vi "AuMT8852B Path Offset Table Read.vi"(5 "Frequency units (Channel)":enum16{"Channel", "MHz"}(ring), 7 "Table (1)":i32=1, 8 "error in (no error)":errorcluster, 11 "VISA session":refnum<visa-resource-name>) -> (0 "error out":errorcluster, 2 "error code":i32, 3 "VISA session out":refnum<visa-resource-name>, 4 "Table values":dbl[][](array[numeric]) format="%.2f")   [LabVIEW 2017]
doc: "Anritsu MT8852B Bluetooth Tester\n\nRetrieves all frequency/offset pairs in a table.\n\nINPUTS\nTable - path offset table (1-10) to use.\nFrequency units - whether the frequencies will be returned as channels or as frequencies in MHz.\n\nOUTPUTS\nTable values - two-dimensional array containing all table frequencies and offsets."
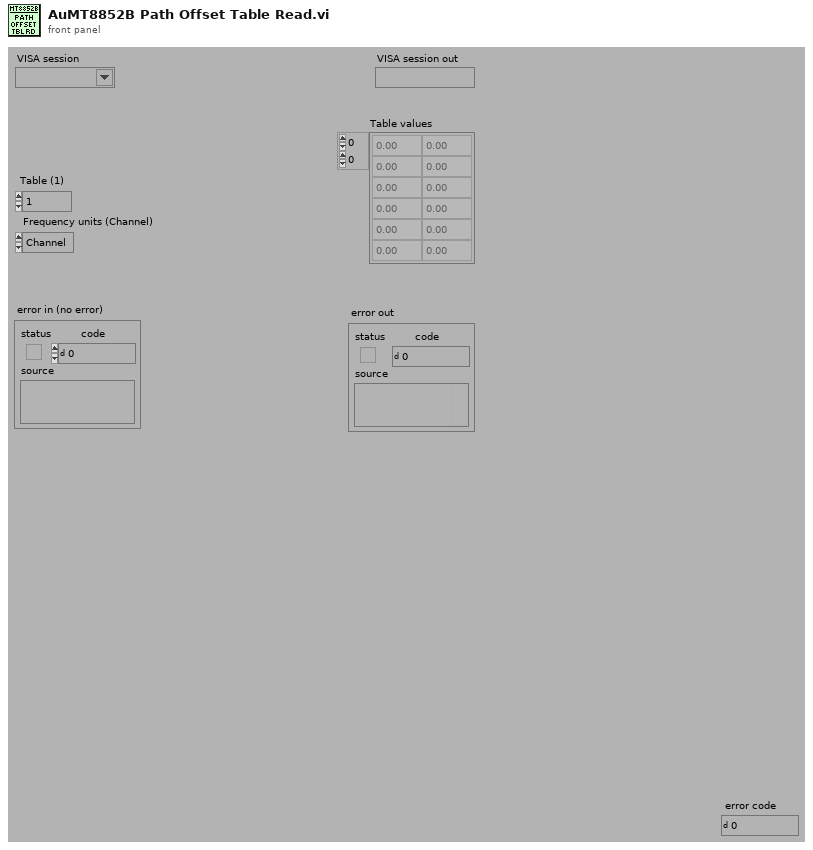
[diagram p1: front panel]
types:
  T1 = enum16{"Simulate", "Range check", "Cache", "Query instrument status"}
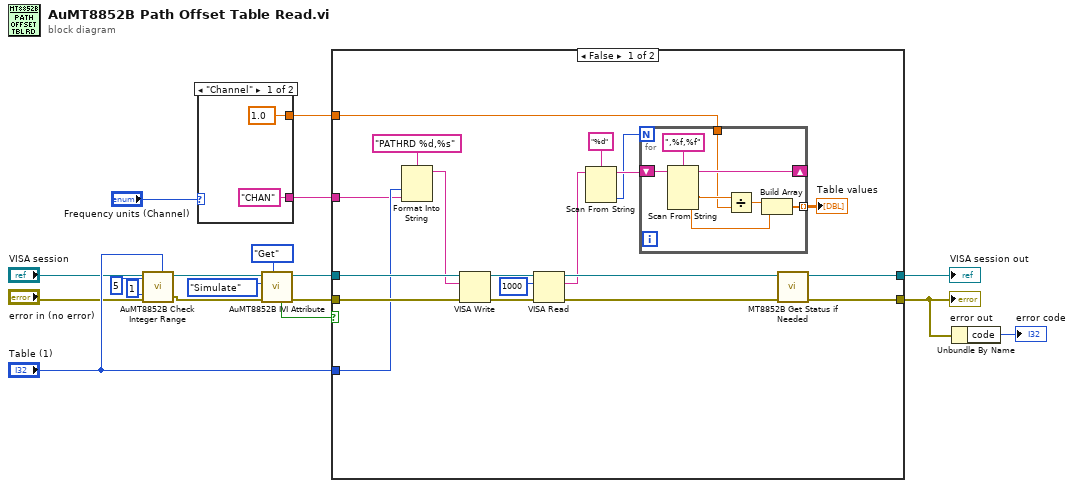
[diagram p0: block diagram]
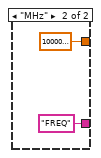
[diagram p2: hidden frame]
diagram:
  n1 = call <instrlib>:"AuMT8852B Check Integer Range.vi"("Value (0)"="Table (1)", "error in (no error)"="error in (no error)", "Lower limit (-1)"=1, "Upper limit (1)"=5, "VISA session"="VISA session") -> ("error out"=w2:errorcluster, "VISA session out"=w3:refnum<visa-resource-name>)  [unwired: 5 in]
  n2 = case shown="\"Channel\"" "Frequency units (Channel)" {
    tunnel: ["CHAN" "FREQ"] -> w4
    tunnel: [1.0 1000000.0] -> w1
    frame "Channel" {
    }
    frame "MHz" {
    }
  }
  n3 = call <instrlib>:"AuMT8852B IVI Attribute.vi"("Set/Get (Set)"=enum16{"Set", "Get"}."Get", "error in (no error)"=w2, "Flag (Simulate)"=T1."Simulate", "VISA session"=w3) -> ("error out"=w16:errorcluster, "VISA session out"=w17:refnum<visa-resource-name>, "Value out"=w13:bool)  [unwired: 5 in]
  n4 = case shown="False" w13 {
    tunnel: [w35 w51] -> w18
    tunnel: [w36 w50] -> w11
    tunnel: w17 -> [w41 w51]
    tunnel: w16 -> [w40 w50]
    tunnel: "Table (1)" -> [w39 _]
    tunnel: w4 -> [w34 _]
    tunnel: w1 -> [w33 _]
    frame False {
      n5 = Format Into String(format string="PATHRD %d,%s" ("Format String"), w39, w34) -> (resulting string=w28:string)  [unwired: 2 in, 1 out]
      n6 = VISA Write(VISA resource name=w41, write buffer=w28, error in (no error)=w40) -> (VISA resource name out=w31:refnum<visa-resource-name>, error out=w32:errorcluster)  [unwired: 1 out]
      n7 = VISA Read(VISA resource name=w31, byte count=u32 1000 ("byte count (0)"), error in (no error)=w32) -> (VISA resource name out=w37:refnum<visa-resource-name>, read buffer=w27:string, error out=w38:errorcluster)  [unwired: 1 out]
      n8 = Scan From String(format string="%d", input string=w27) -> (remaining string=w26:string, output 1=w24:i32)  [unwired: 3 in, 2 out]
      n9 = for {
        N: w24 -> [_]
        shift-right: [w47] -> _
        shift-left: w26 -> [w48]
        tunnel: w33 -> [w45]
        tunnel: [w42] -> w23 mode=indexing
        n10 = Scan From String(format string=",%f,%f", input string=w48) -> (remaining string=w47:string, output 1=w46:dbl, output 2=w43:dbl)  [unwired: 4 in, 2 out]
        n11 = Divide(x=w46, y=w45) -> (x/y=w44:dbl)
        n12 = Build Array(w44, w43) -> (w42:dbl[])
      }
      "Table values" <- w23
      n13 = call <instrlib>:"MT8852B Get Status if Needed.vi"("error in (no error)"=w38, "VISA session"=w37) -> ("error out"=w36:errorcluster, "VISA session out"=w35:refnum<visa-resource-name>)  [unwired: 8 in]
    }
    frame True {
      (unwired) "" ("Response")
    }
  }
  "error out" <- w11
  "VISA session out" <- w18
  n14 = Unbundle By Name(w11) -> ("code"=→"error code":i32)
